vi "findCOM.vi"(1 "error in (no error)":errorcluster) -> (3 "错误输出":errorcluster, 4 "COM out":string)   [LabVIEW 2018]
uses:
  <vilib>/Instr/_visa.llb/VISA Configure Serial Port (Instr).vi
  <vilib>/regexp/Match Regular Expression.xnode
panel:
  out "读取缓冲区":string
  out "数组":string[](array[string])
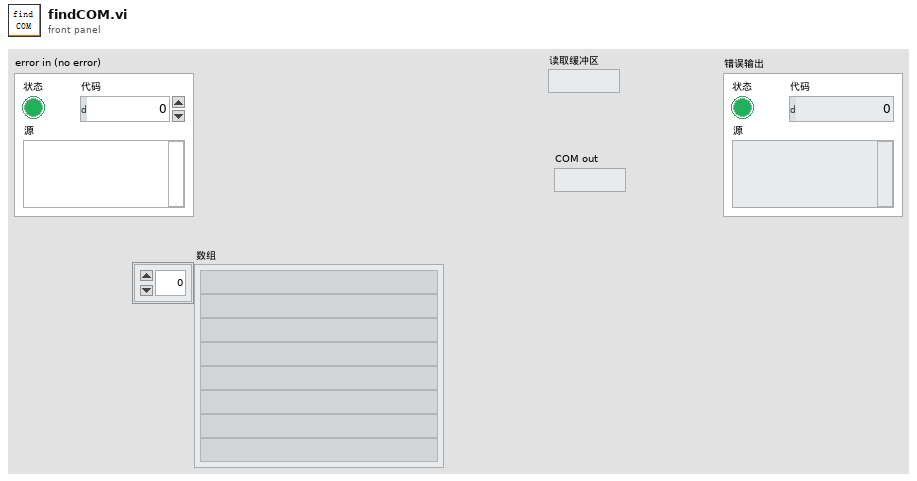
[diagram p1: front panel]
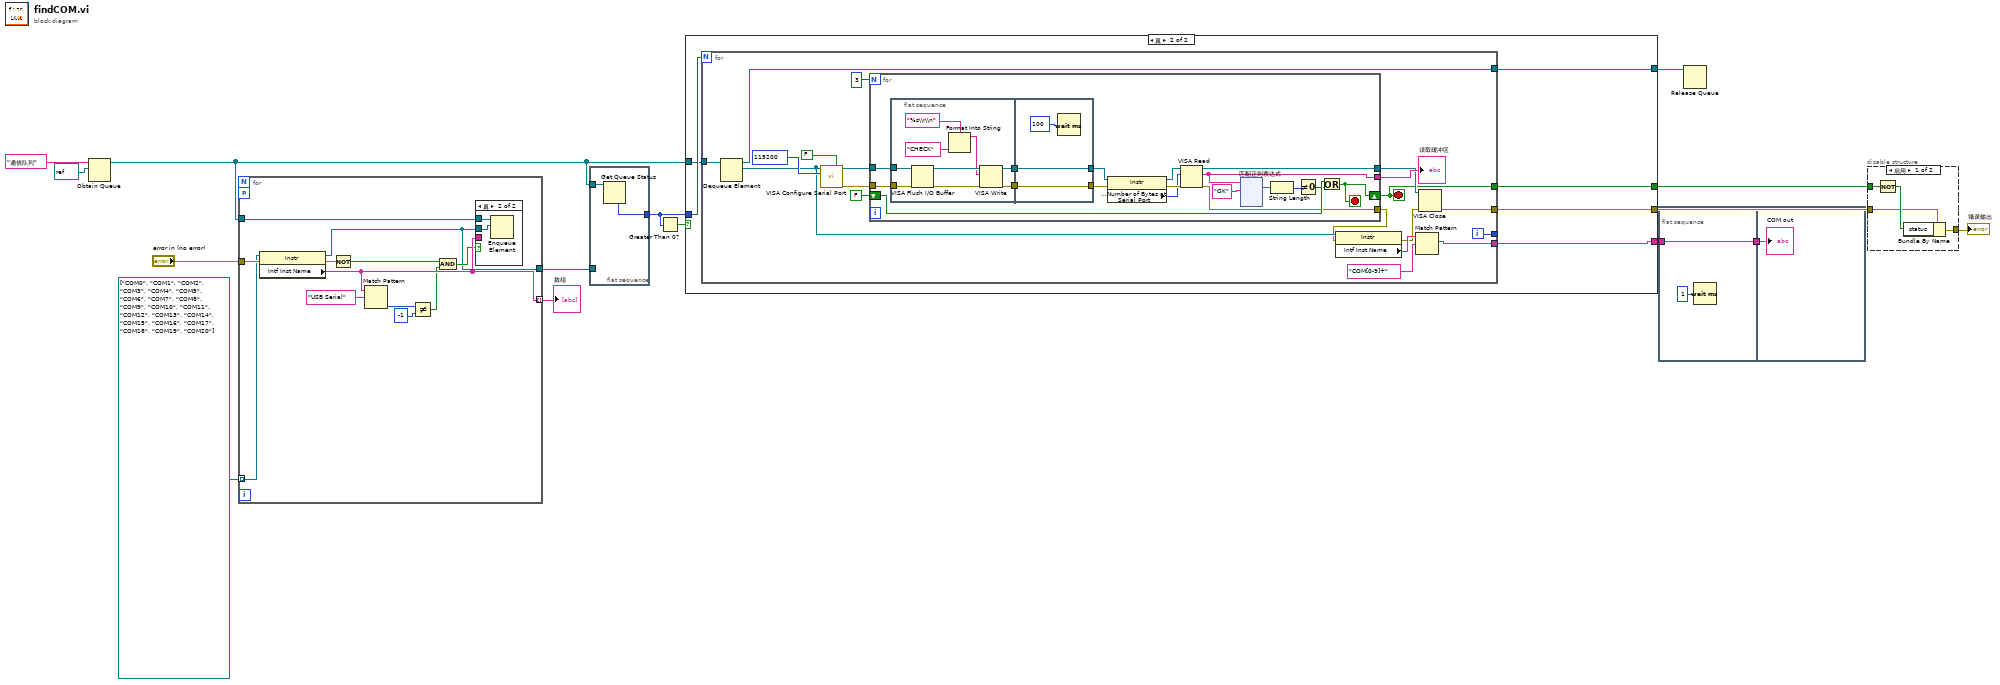
[diagram p0: block diagram]
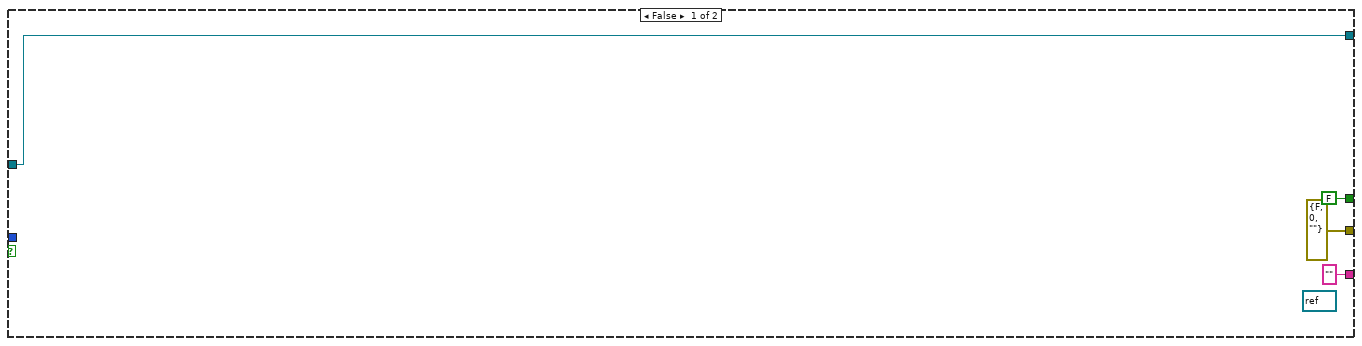
[diagram p2: hidden frame]
diagram:
  n1 = Obtain Queue(name (unnamed)="通信队列" ("名称（未命名）"), element data type=refnum<visa-resource-name> refnum ("引用")) -> (queue out=w9:refnum<queue>)  [unwired: 3 in, 2 out]
  n2 = for {
    tunnel: refnum<visa-resource-name>[] ["COM0", "COM1", "COM2", "COM3", "COM4", "COM5", "COM6", "COM7", "COM8", "COM9", "COM10", "COM11", "COM12", "COM13", "COM14", "COM15", "COM16", "COM17", "COM18", "COM19", "COM20"] ("添加的数组") -> [w26] mode=indexing
    tunnel: "error in (no error)" -> [w27]
    tunnel: [w16] -> w10
    tunnel: [w21] -> w13 mode=indexing
    workers-P: _ -> [_]
    tunnel: w9 -> [w17]
    n3 = property class="Instr"(reference=w26, error in=w27) -> (reference out=w16:refnum<visa-resource-name>, error out=w23:errorcluster, "Intf Inst Name"=w21:string)
    n4 = Not(x=w23) -> (.not. x?=w20:bool)
    n5 = Match Pattern(string=w21, regular expression="USB Serial" ("正则表达式")) -> (offset past match=w25:i32)  [unwired: 1 in, 3 out]
    n6 = Not Equal?(x=w25, y=-1) -> (x != y?=w19:bool)
    n7 = And(x=w20, y=w19) -> (x .and. y?=w18:bool)
    n8 = case shown="真" w18 {
      tunnel: w21 -> [_ _]
      tunnel: w17 -> [_ w29]
      tunnel: w16 -> [_ w28]
      frame False {
      }
      frame True {
        n9 = Enqueue Element(queue=w29, element=w28) -> ()  [unwired: 2 in, 3 out]
      }
    }
  }
  "数组" <- w13
  n10 = flat-sequence {
    tunnel: w10 -> [_]
    tunnel: w9 -> [w31]
    tunnel: [w30] -> w4
    frame #0 {
      n11 = Get Queue Status(queue=w31) -> (# elements in queue=w30:i32)  [unwired: 2 in, 7 out]
    }
  }
  n12 = Greater Than 0?(x=w4) -> (x > 0?=w3:bool)
  n13 = case shown="真" w3 {
    tunnel: w4 -> [_ w41]
    tunnel: w9 -> [w35 w40]
    tunnel: [w35 w39] -> w8
    tunnel: [errorcluster {"status"=FALSE, "code"=0, "source"=""} ("error out") w38] -> w7
    tunnel: [FALSE w37] -> w5
    tunnel: ["" ("Intf Inst Name") w36] -> w2
    frame False {
      (unwired) refnum<visa-resource-name> refnum ("引用")
    }
    frame True {
      n14 = for {
        N: w41 -> [_]
        tunnel: w40 -> [w60]
        tunnel: [w51] -> w37
        tunnel: [w50] -> _
        tunnel: [w49] -> w39
        tunnel: [w48] -> w38
        tunnel: [w45] -> w36
        i -> [w50]
        stop <- w51 stop-if-true
        n15 = Dequeue Element(queue=w60) -> (queue out=w49:refnum<queue>, element=w44:refnum<visa-resource-name>)  [unwired: 2 in, 2 out]
        n16 = call-poly "VISA Configure Serial Port"("VISA resource name"=w44, "Enable Termination\nChar (T)"=FALSE ("Enable Termination\nChar (T)"), "baud rate (9600)"=u32 115200) -> ("VISA resource name out"=w56:refnum<visa-resource-name>, "error out"=w55:errorcluster)  [unwired: 11 in]
        n17 = for {
          N: 3 -> [_]
          tunnel: w56 -> [w78]
          tunnel: w55 -> [w77]
          tunnel: [w69] -> w54
          shift-right: [w64] -> w51
          shift-left: FALSE -> [w67]
          tunnel: [w66] -> w52
          tunnel: [w65] -> w43
          stop <- w64 stop-if-true
          n18 = flat-sequence {
            tunnel: w78 -> [w200]
            tunnel: w77 -> [w199]
            tunnel: [w197] -> w71
            tunnel: [w196] -> w70
            tunnel: [w203] -> w74
            tunnel: [w204] -> w76
            tunnel: w71 -> [w204]
            tunnel: w70 -> [w203]
            frame #0 {
              n19 = VISA Flush I/O Buffer(VISA resource name=w200, error in (no error)=w199) -> (VISA resource name out=w201:refnum<visa-resource-name>, error out=w198:errorcluster)  [unwired: 1 in]
              n20 = Format Into String(format string="%s\\r\\n" ("格式字符串"), "CHECK" ("写入缓冲区")) -> (resulting string=w193:string)  [unwired: 2 in, 1 out]
              n21 = VISA Write(VISA resource name=w201, write buffer=w193, error in (no error)=w198) -> (VISA resource name out=w197:refnum<visa-resource-name>, error out=w196:errorcluster)  [unwired: 1 out]
            }
            frame #1 {
              n22 = Wait (ms)(milliseconds to wait=u32 100 ("等待时间（毫秒）")) -> ()  [unwired: 1 out]
            }
          }
          n23 = property class="Instr"(reference=w76, error in=w74) -> (reference out=w75:refnum<visa-resource-name>, error out=w73:errorcluster, "Serial Settings:Number of Bytes at Serial Port"=w72:u32)
          n24 = VISA Read(VISA resource name=w75, byte count=w72, error in (no error)=w73) -> (VISA resource name out=w66:refnum<visa-resource-name>, read buffer=w69:string, error out=w65:errorcluster)  [unwired: 1 out]
          n25 = xnode "匹配正则表达式"("输入字符串"=w69, "正则表达式"="OK") -> ("所有匹配"=w63:string)  [unwired: 4 in, 4 out]
          n26 = String Length(string=w63) -> (length=w62:i32)
          n27 = Not Equal To 0?(x=w62) -> (x != 0?=w61:bool)
          n28 = Or(x=w67, y=w61) -> (x .or. y?=w64:bool)
        }
        "读取缓冲区" <- w54
        n29 = property class="Instr"(reference=w44, error in=w43) -> (error out=w42:errorcluster, "Intf Inst Name"=w47:string)  [unwired: 1 out]
        n30 = Match Pattern(string=w47, regular expression="COM[0-9]+" ("正则表达式")) -> (match substring=w45:string)  [unwired: 1 in, 3 out]
        n31 = VISA Close(VISA resource name=w52, error in (no error)=w42) -> (error out=w48:errorcluster)
      }
    }
  }
  n32 = flat-sequence {
    tunnel: w2 -> [w206]
    tunnel: [w206] -> w1
    tunnel: w1 -> [w207]
    frame #0 {
      n33 = Wait (ms)(milliseconds to wait=u32 1 ("等待时间（毫秒）")) -> ()  [unwired: 1 out]
    }
    frame #1 {
      "COM out" <- w207
    }
  }
  n34 = Release Queue(queue=w8) -> ()  [unwired: 2 in, 3 out]
  n35 = disable-structure shown="启用" {
    disable-tunnel: w7 -> [w210 _]
    disable-tunnel: [w209 _] -> w6
    disable-tunnel: w5 -> [w208 _]
    frame Enabled {
      n36 = Not(x=w208) -> (.not. x?=w211:bool)
      n37 = Bundle By Name(cluster=w210, "status"=w211) -> (w209:errorcluster)
    }
    frame Disabled {
    }
  }
  "错误输出" <- w6
